vi "Convert TimeStamp To Raw Time.vi"(0 "error in (no error)":errorcluster, 1 "time stamp":timestamp) -> (2 "error in (no error) 2":errorcluster, 3 "Nanoseconds":u32, 4 "Seconds":u32)   [LabVIEW 2015]
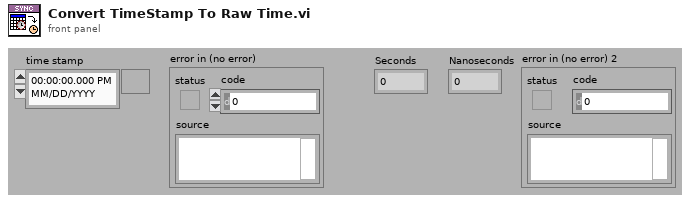
[diagram p1: front panel]
types:
  T1 = cluster{"high":i32, "mid high":u32, "mid low":u32, "low":u32}
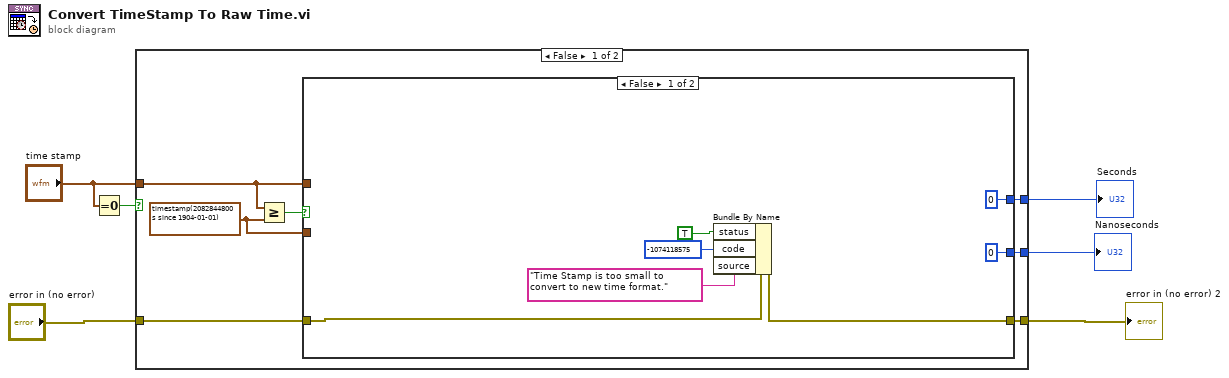
[diagram p0: block diagram]
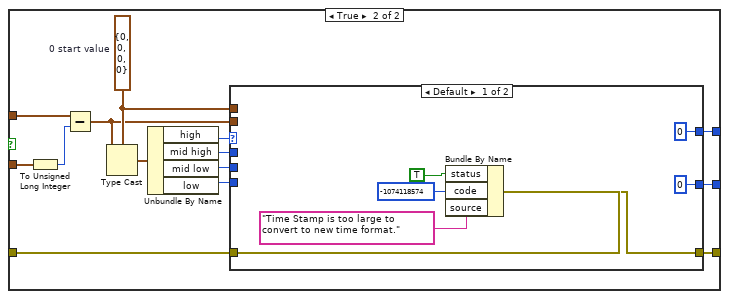
[diagram p2: hidden frame]
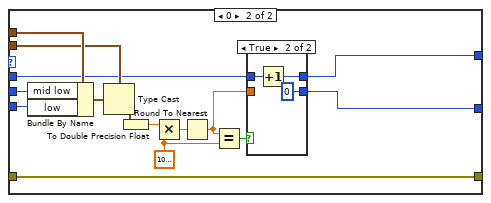
[diagram p3: hidden frame]
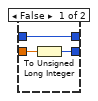
[diagram p4: hidden frame]
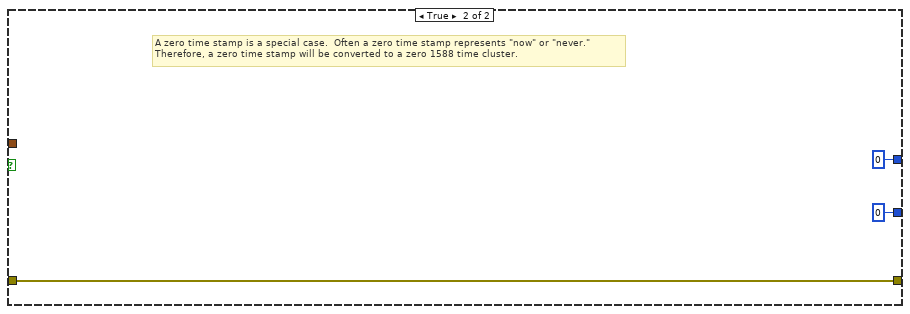
[diagram p5: hidden frame]
diagram:
  n1 = Equal To 0?(x="time stamp") -> (x = 0?=w3:bool)
  n2 = case shown="False" w3 {
    tunnel: [w13 w65] -> w1
    tunnel: "error in (no error)" -> [w12 w65]
    tunnel: "time stamp" -> [w10 _]
    tunnel: [w8 u32 0 ("mid high")] -> w5
    tunnel: [w7 u32 0] -> w6
    frame False {
      w9 = timestamp(2082844800 s since 1904-01-01) ("x+y")
      n3 = Greater Or Equal?(x=w10, y=w9) -> (x >= y?=w11:bool)
      n4 = case shown="False" w11 {
        tunnel: [w17 w28] -> w13
        tunnel: w12 -> [w16 w27]
        tunnel: w10 -> [_ w24]
        tunnel: w9 -> [_ w23]
        tunnel: [u32 0 ("mid high") w22] -> w8
        tunnel: [u32 0 w21] -> w7
        frame False {
          n5 = Bundle By Name(cluster=w16, "status"=TRUE, "code"=-1074118575, "source"="Time Stamp is too small to convert to new time format.") -> (w17:errorcluster)
        }
        frame True {
          w31 = T1 {"high"=0, "mid high"=0, "mid low"=0, "low"=0}  # 0 start value
          n6 = To Unsigned Long Integer(number=w23) -> (unsigned 32bit integer=w26:u32)
          n7 = Subtract(x=w24, y=w26) -> (x-y=w25:timestamp)
          n8 = Type Cast(type=w31, x=w25) -> (*(type *) &x=w34:T1)
          n9 = Unbundle By Name(w34) -> ("high"=w32:i32, "mid high"=w33:u32, "mid low"=w30:u32, "low"=w29:u32)
          n10 = case shown="Default" w32 {
            tunnel: w33 -> [_ w45]
            tunnel: w27 -> [w41 w48]
            tunnel: w31 -> [_ w56]
            tunnel: w30 -> [_ w55]
            tunnel: w29 -> [_ w54]
            tunnel: w25 -> [_ w52]
            tunnel: [w40 w48] -> w28
            tunnel: [u32 0 ("mid high") w43] -> w22
            tunnel: [u32 0 w42] -> w21
            frame Default {
              n11 = Bundle By Name(cluster=w41, "status"=TRUE, "code"=-1074118574, "source"="Time Stamp is too large to convert to new time format.") -> (w40:errorcluster)
            }
            frame 0 {
              w47 = 1000000000.0
              n12 = Bundle By Name(cluster=w56, "mid low"=w55, "low"=w54) -> (w53:T1)
              n13 = Type Cast(type=w52, x=w53) -> (*(type *) &x=w50:timestamp)
              n14 = To Double Precision Float(number=w50) -> (double precision float=w49:dbl)
              n15 = Multiply(x=w49, y=w47) -> (x*y=w51:dbl)
              n16 = Round To Nearest(number=w51) -> (nearest integer value=w44:dbl)
              n17 = Equal?(x=w44, y=w47) -> (x = y?=w46:bool)
              n18 = case shown="True" w46 {
                tunnel: w45 -> [w57 w62]
                tunnel: w44 -> [w59 _]
                tunnel: [w58 u32 0] -> w42
                tunnel: [w57 w61] -> w43
                frame False {
                  n19 = To Unsigned Long Integer(number=w59) -> (unsigned 32bit integer=w58:u32)
                }
                frame True {
                  n20 = Increment(x=w62) -> (x+1=w61:u32)
                }
              }
            }
          }
        }
      }
    }
    frame True {
      # "A zero time stamp is a special case.  Often a zero time stamp represents \"now\" or \"never.\"\nTherefore, a zero time stamp will be converted to a zero 1588 time cluster."
    }
  }
  "Nanoseconds" <- w6
  "Seconds" <- w5
  "error in (no error) 2" <- w1
